vi "Configure Module.vi"(8 "error in":errorcluster, 10 "IOV ref in":refnum<k21>, 11 "9226 in":refnum<class "9226.lvclass">) -> (0 "error out":errorcluster, 2 "IOV ref out":refnum<k21>, 3 "9226 out":refnum<class "9226.lvclass">)   [LabVIEW 2017, in "Modules.lvlib" / "9226.lvclass"]
uses:
  9226.lvclass
  9226.lvclass/9226.ctl
  <resource>/objmgr/cRIO.rc
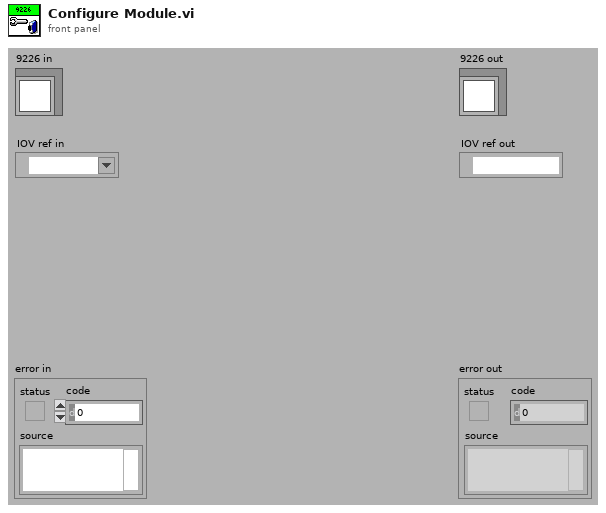
[diagram p1: front panel]
types:
  T1 = typedef "Modules.lvlib/9226.lvclass/Supported RTD Types.ctl" = u32
  T2 = cluster{"Ohm degree range":u32, "RTD type":T1, "RTD user-defined A constant":dbl, "RTD user-defined B constant":dbl, "RTD user-defined C constant":dbl, "RTD user-defined Ro constant":dbl}[]
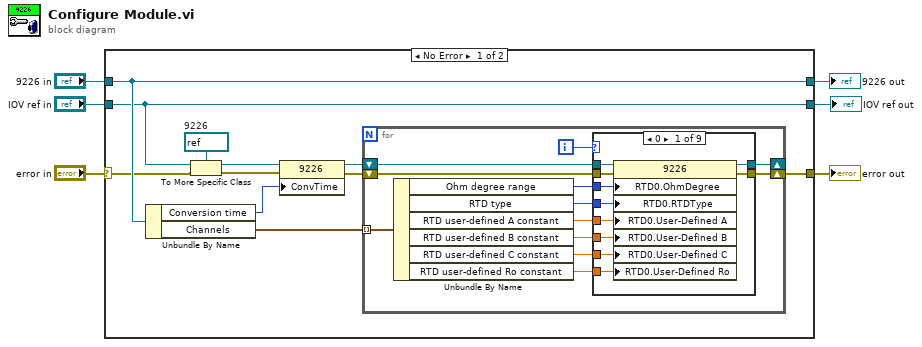
[diagram p0: block diagram]
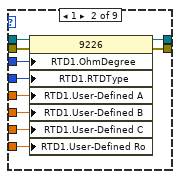
[diagram p2: hidden frame]
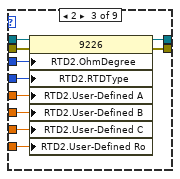
[diagram p3: hidden frame]
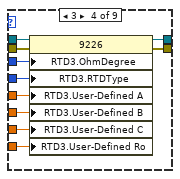
[diagram p4: hidden frame]
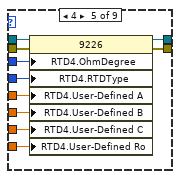
[diagram p5: hidden frame]
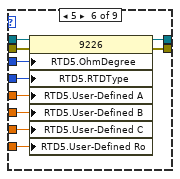
[diagram p6: hidden frame]
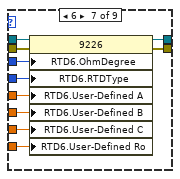
[diagram p7: hidden frame]
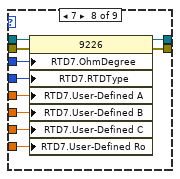
[diagram p8: hidden frame]
diagram:
  n1 = case shown="No Error" "error in" {
    selector: "error in" -> [w7 w114]
    tunnel: [w15 w114] -> w5
    tunnel: [w17 w113] -> w3
    tunnel: "9226 in" -> [w17 w113]
    tunnel: "IOV ref in" -> [w14 w112]
    tunnel: [w14 w112] -> w1
    frame No Error {
      w16 = refnum<k21> refnum  # 9226
      n2 = Unbundle By Name(w17) -> ("Conversion time"=w13:u32, "Channels"=w8:T2)
      n3 = To More Specific Class(target class=w16, reference=w14, error in=w7) -> (specific class reference=w12:refnum<k21>, error out=w11:errorcluster)
      n4 = property class="9226"(reference=w12, error in=w11, "ConvTime"=w13) -> (reference out=w9:refnum<k21>, error out=w10:errorcluster)
      n5 = for {
        shift-right: [w29] -> w15
        shift-left: w10 -> [w22]
        shift-right: [w20] -> _
        shift-left: w9 -> [w21]
        tunnel: w8 -> [w19] mode=indexing
        i -> [w18]
        n6 = Unbundle By Name(w19) -> ("Ohm degree range"=w28:u32, "RTD type"=w27:T1, "RTD user-defined A constant"=w26:dbl, "RTD user-defined B constant"=w25:dbl, "RTD user-defined C constant"=w24:dbl, "RTD user-defined Ro constant"=w23:dbl)
        n7 = case shown="0" w18 {
          tunnel: [w39 w49 w59 w69 w79 w89 w99 w109 w110] -> w29
          tunnel: w28 -> [w38 w48 w58 w68 w78 w88 w98 w108 _]
          tunnel: w27 -> [w37 w40 w50 w60 w74 w80 w90 w100 _]
          tunnel: w26 -> [w36 w41 w51 w61 w73 w81 w91 w101 _]
          tunnel: w25 -> [w35 w42 w52 w62 w72 w82 w92 w102 _]
          tunnel: w24 -> [w34 w43 w53 w63 w71 w83 w93 w103 _]
          tunnel: w23 -> [w33 w44 w54 w64 w70 w84 w94 w104 _]
          tunnel: w22 -> [w32 w47 w57 w67 w77 w87 w97 w107 w110]
          tunnel: w21 -> [w31 w46 w56 w66 w76 w86 w96 w106 w111]
          tunnel: [w30 w45 w55 w65 w75 w85 w95 w105 w111] -> w20
          frame 0 {
            n8 = property class="9226"(reference=w31, error in=w32, "RTD0.OhmDegree"=w38, "RTD0.RTDType"=w37, "RTD0.User-Defined A"=w36, "RTD0.User-Defined B"=w35, "RTD0.User-Defined C"=w34, "RTD0.User-Defined Ro"=w33) -> (reference out=w30:refnum<k21>, error out=w39:errorcluster)
          }
          frame 1 {
            n9 = property class="9226"(reference=w46, error in=w47, "RTD1.OhmDegree"=w48, "RTD1.RTDType"=w40, "RTD1.User-Defined A"=w41, "RTD1.User-Defined B"=w42, "RTD1.User-Defined C"=w43, "RTD1.User-Defined Ro"=w44) -> (reference out=w45:refnum<k21>, error out=w49:errorcluster)
          }
          frame 2 {
            n10 = property class="9226"(reference=w56, error in=w57, "RTD2.OhmDegree"=w58, "RTD2.RTDType"=w50, "RTD2.User-Defined A"=w51, "RTD2.User-Defined B"=w52, "RTD2.User-Defined C"=w53, "RTD2.User-Defined Ro"=w54) -> (reference out=w55:refnum<k21>, error out=w59:errorcluster)
          }
          frame 3 {
            n11 = property class="9226"(reference=w66, error in=w67, "RTD3.OhmDegree"=w68, "RTD3.RTDType"=w60, "RTD3.User-Defined A"=w61, "RTD3.User-Defined B"=w62, "RTD3.User-Defined C"=w63, "RTD3.User-Defined Ro"=w64) -> (reference out=w65:refnum<k21>, error out=w69:errorcluster)
          }
          frame 4 {
            n12 = property class="9226"(reference=w76, error in=w77, "RTD4.OhmDegree"=w78, "RTD4.RTDType"=w74, "RTD4.User-Defined A"=w73, "RTD4.User-Defined B"=w72, "RTD4.User-Defined C"=w71, "RTD4.User-Defined Ro"=w70) -> (reference out=w75:refnum<k21>, error out=w79:errorcluster)
          }
          frame 5 {
            n13 = property class="9226"(reference=w86, error in=w87, "RTD5.OhmDegree"=w88, "RTD5.RTDType"=w80, "RTD5.User-Defined A"=w81, "RTD5.User-Defined B"=w82, "RTD5.User-Defined C"=w83, "RTD5.User-Defined Ro"=w84) -> (reference out=w85:refnum<k21>, error out=w89:errorcluster)
          }
          frame 6 {
            n14 = property class="9226"(reference=w96, error in=w97, "RTD6.OhmDegree"=w98, "RTD6.RTDType"=w90, "RTD6.User-Defined A"=w91, "RTD6.User-Defined B"=w92, "RTD6.User-Defined C"=w93, "RTD6.User-Defined Ro"=w94) -> (reference out=w95:refnum<k21>, error out=w99:errorcluster)
          }
          frame 7 {
            n15 = property class="9226"(reference=w106, error in=w107, "RTD7.OhmDegree"=w108, "RTD7.RTDType"=w100, "RTD7.User-Defined A"=w101, "RTD7.User-Defined B"=w102, "RTD7.User-Defined C"=w103, "RTD7.User-Defined Ro"=w104) -> (reference out=w105:refnum<k21>, error out=w109:errorcluster)
          }
          frame Default {
          }
        }
      }
    }
    frame Error {
    }
  }
  "error out" <- w5
  "9226 out" <- w3
  "IOV ref out" <- w1
